vi "OleDB.vi"() -> ()   [LabVIEW 2012]
uses:
  OleDBClass/OleDBClass.lvclass
  System.Windows.Forms
panel:
  in  "停止":bool
  in  "DataGridView":refnum<k24>(container)
  in  "cmdText":string="Select * from fetchdata"
  in  "connectionString":string="Provider=Microsoft.Jet.OLEDB.4.0;Data Source=E:\\BOOK\\功能块\\NET工具\\数据库\\OleDB\\OleDBClass\\LabVIEW.mdb;Persist Security Info=False"
  out "error out":errorcluster caption="错误输出"
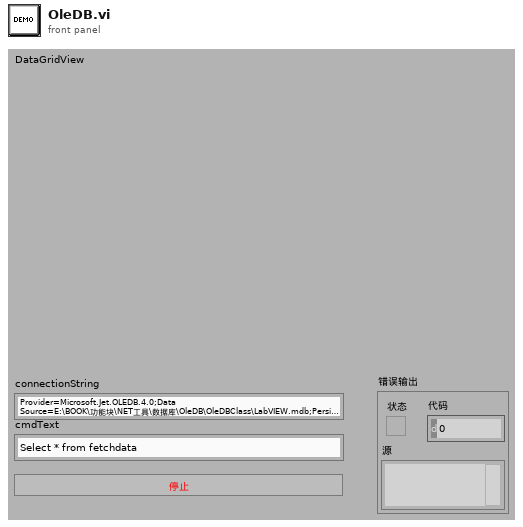
[diagram p1: front panel]
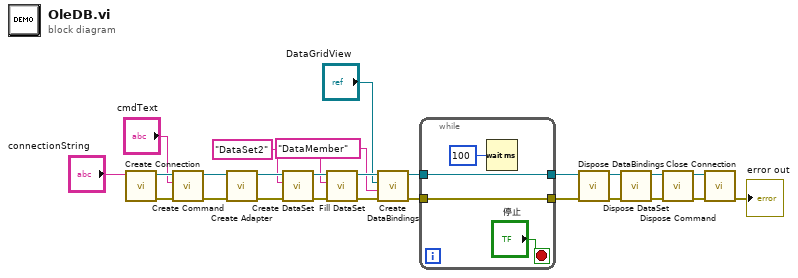
[diagram p0: block diagram]
diagram:
  w5 = "DataMember" ("srcTable")
  n1 = call "Create Connection.vi"("connectionString"="connectionString") -> ("error out"=w24:errorcluster, "OleDBClass 输出"=w25:refnum<class "OleDBClass.lvclass">)  [unwired: 9 in]
  n2 = call "Create Command.vi"("error in (no error)"=w24, "cmdText"="cmdText", "OleDBClass 输入"=w25) -> ("error out"=w18:errorcluster, "OleDBClass 输出"=w19:refnum<class "OleDBClass.lvclass">)  [unwired: 7 in]
  n3 = call "Create Adapter.vi"("error in (no error)"=w18, "OleDBClass 输入"=w19) -> ("error out"=w16:errorcluster, "OleDBClass 输出"=w17:refnum<class "OleDBClass.lvclass">)  [unwired: 8 in]
  n4 = call "Create DataSet.vi"("error in (no error)"=w16, "dataSetName"="DataSet2", "OleDBClass 输入"=w17) -> ("error out"=w13:errorcluster, "OleDBClass 输出"=w14:refnum<class "OleDBClass.lvclass">)  [unwired: 7 in]
  n5 = call "Fill DataSet.vi"("error in (no error)"=w13, "srcTable"=w5, "OleDBClass 输入"=w14) -> ("error out"=w9:errorcluster, "OleDBClass 输出"=w10:refnum<class "OleDBClass.lvclass">)  [unwired: 7 in]
  n6 = call "Create DataBindings.vi"("error in (no error)"=w9, "DataMember"=w5, "DataGridView"="DataGridView", "OleDBClass 输入"=w10) -> ("error out"=w8:errorcluster, "OleDBClass 输出"=w7:refnum<class "OleDBClass.lvclass">)  [unwired: 6 in]
  n7 = while {
    tunnel: w7 -> [w28]
    tunnel: [w28] -> w4
    tunnel: w8 -> [w27]
    tunnel: [w27] -> w2
    stop <- "停止" stop-if-true
    n8 = Wait (ms)(milliseconds to wait=u32 100 ("等待时间（毫秒）")) -> ()  [unwired: 1 out]
  }
  n9 = call "Dispose DataBindings.vi"("error in (no error)"=w2, "OleDBClass 输入"=w4) -> ("error out"=w1:errorcluster, "OleDBClass 输出"=w3:refnum<class "OleDBClass.lvclass">)  [unwired: 8 in]
  n10 = call "Dispose DataSet.vi"("error in (no error)"=w1, "OleDBClass 输入"=w3) -> ("error out"=w11:errorcluster, "OleDBClass 输出"=w12:refnum<class "OleDBClass.lvclass">)  [unwired: 8 in]
  n11 = call "Dispose Command.vi"("error in (no error)"=w11, "OleDBClass 输入"=w12) -> ("error out"=w22:errorcluster, "OleDBClass 输出"=w23:refnum<class "OleDBClass.lvclass">)  [unwired: 8 in]
  n12 = call "Close Connection.vi"("error in (no error)"=w22, "OleDBClass 输入"=w23) -> ("error out"=→"error out":errorcluster)  [unwired: 8 in, 1 out]
